vi "Build_array.vi"(0 "Min Amplitude":dbl=3.0, 1 "Max Amplitude":dbl=6.0, 2 "Amplitude Delta":dbl=1.0, 3 "Min Frequency":dbl=3.0, 4 "Max Frequency":dbl=6.0, 5 "Frequency Delta":dbl=1.0) -> (14 "Amplitudes":dbl[](array[numeric]), 19 "Frequencies":dbl[](array[numeric]))   [LabVIEW 2010]
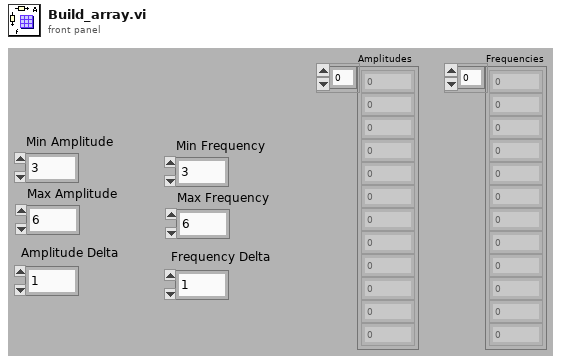
[diagram p1: front panel]
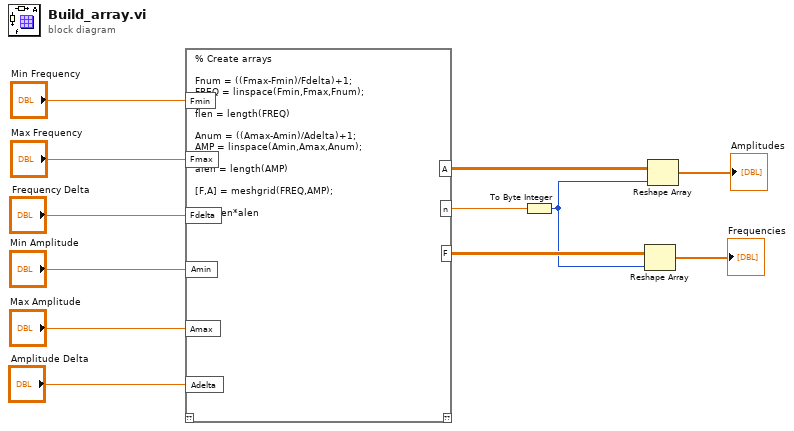
[diagram p0: block diagram]
diagram:
  n1 = script code="% Create arrays\n\nFnum = ((Fmax-Fmin)/Fdelta)+1;\nFREQ = linspace(Fmin,Fmax,Fnum);\n\nflen = length(FREQ)\n\nAnum = ((Amax-Amin)/Adelta)+1;\nAMP = linspace(Amin,Amax,Anum);\n\nalen = length(AMP)\n\n[F,A] = meshgrid(FREQ,AMP);\n\nn = flen*alen"("Fmin"="Min Frequency", "Fmax"="Max Frequency", "Fdelta"="Frequency Delta", "Amin"="Min Amplitude", "Amax"="Max Amplitude", "Adelta"="Amplitude Delta") -> ("A"=w6:dbl[][], "F"=w3:dbl[][], "n"=w2:dbl)  [unwired: 1 in, 1 out]
  n2 = To Byte Integer(number=w2) -> (8bit integer=w1:i8)
  n3 = Reshape Array(w3, w1) -> (→"Frequencies":dbl[])
  n4 = Reshape Array(w6, w1) -> (→"Amplitudes":dbl[])
